vi "SignalGenerator.vi"() -> ()   [LabVIEW 2016]
doc: "I. Description:\nThis example demonstrates how to continuously output a waveform using an internal sample clock. The automatic regeneration of data has been disabled, so new data has to be provided throughout the duration of the continuous Analog Output operation. This allows the generation of any arbitrary frequency as this VI computes new data for each iteration of the loop, maintaining phase continuity of the signal. The regeneration of data has also been adjusted so that the newest data is output as quickly as possible; thus reducing the lag between the changing of the data and the output of that data.\n\nII. Instructions for Running:\n1. Select the Physical Channel to correspond to where your signal is output on the DAQ device.\n2. Enter the Minimum and Maximum Voltage range.\n3. Specify the desired Sample Clock Rate of the output Waveform. Higher sample clock rates will produce a smoother waveform.\n4. Manually specify the Analog Output buffer size, in number of samples. A larger buffer would help non-regenerative operations avoid errors due to occasional high CPU load. \nNote: \nThe Analog Output buffer has to be at least as big as the amount of data being written to the board per iteration. The recommended buffer size would be at least twice the amount of data being written to the board per iteration.\n5. Enter the Waveform Information. See the documentation of the Basic Function Generator SubVI for information on each parameter.\n\nIII. Block Diagram Steps:\n1. Create an Analog Output Voltage channel.\n2. Configure the task to prohibit the automatic regeneration of data.\n2a. Set the transfer condition to Less than Full. Allows for more rapid updates of Output Buffer.\n3. Call the DAQmx (Sample Clock) VI to set the sample clock rate. Additionally, set the sample mode to Continuous.\n4. Read the actual sample clock rate (eventually coerced depending on the hardware used). \n5. Compute the desired waveform, using the buffer size and the actual update rate. This VI keeps track of the phase of the waveform to ensure that the generated signal is continuous.\n6. Write the waveform to the output buffer. \n7a. Call the Start VI. This is only needed when the loop is executed for the first time.\n7b. Do nothing.\n8. Loop continuously until user presses the Stop button. Every iteration computes and writes a new waveform to the buffer.\n9. Call the Clear Task VI to clear the Task.\n10. Use the popup dialog box to display an error or warning if any.\n\nIV. I/O Connections Overview:\nMake sure your signal output terminal matches the Physical Channel I/O Control. For further connection information, refer to your hardware reference manual."
uses:
  <vilib>/Utility/error.llb/DialogType.ctl
  <vilib>/DAQmx/write.llb/DAQmx Write.vi
  <vilib>/DAQmx/create/channels.llb/DAQmx Create Virtual Channel.vi
  <vilib>/DAQmx/configure/timing.llb/DAQmx Timing.vi
  <vilib>/DAQmx/miscellaneous.llb/DAQmx Fill In Error Info.vi
  <vilib>/measure/NI_MABase.lvlib
  <resource>/objmgr/daqmx.rc
panel:
  in  "Size (Samples)":u32=10000
  out "Actual Sample Clock Rate":dbl=20000.0 format="%.2f"
  in  "Sample Clock Rate":dbl=10000.0 format="%0.2f"
  in  "Waveform Type":T1(ring)
  in  "Frequency":dbl=10.0 format="%.2f"
  in  "Amplitude":dbl=0.1 format="%0.2p"
  out "Waveform Graph":waveform(dbl)(graph)={"t0"=timestamp(12.75 s since 1904-01-01), "dt"=5e-05, "Y"=[]} caption="Output Waveform"
  in  "Physical Channels":tag="DAQ/ao0"
  in  "Minimum Value":dbl=-1.0 format="%0.2f"
  in  "Maximum Value":dbl=1.0 format="%0.2f"
  in  "stop":bool
  # "For instructions, select Help>>Show Context Help"
  # "Channel Parameters"
  # "Timing Parameters"
  # "Buffer Parameters"
  # "Waveform Information"
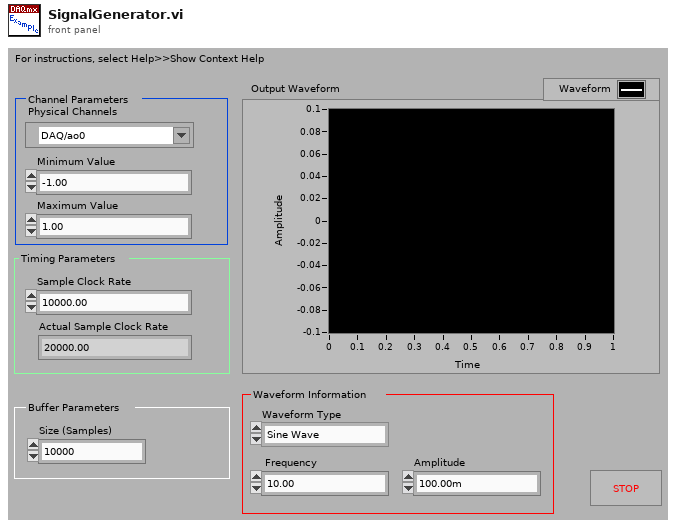
[diagram p1: front panel]
types:
  T1 = enum16{"Sine Wave", "Triangle Wave", "Square Wave", "Sawtooth Wave"}
  T2 = typedef "DialogType.ctl" = u16
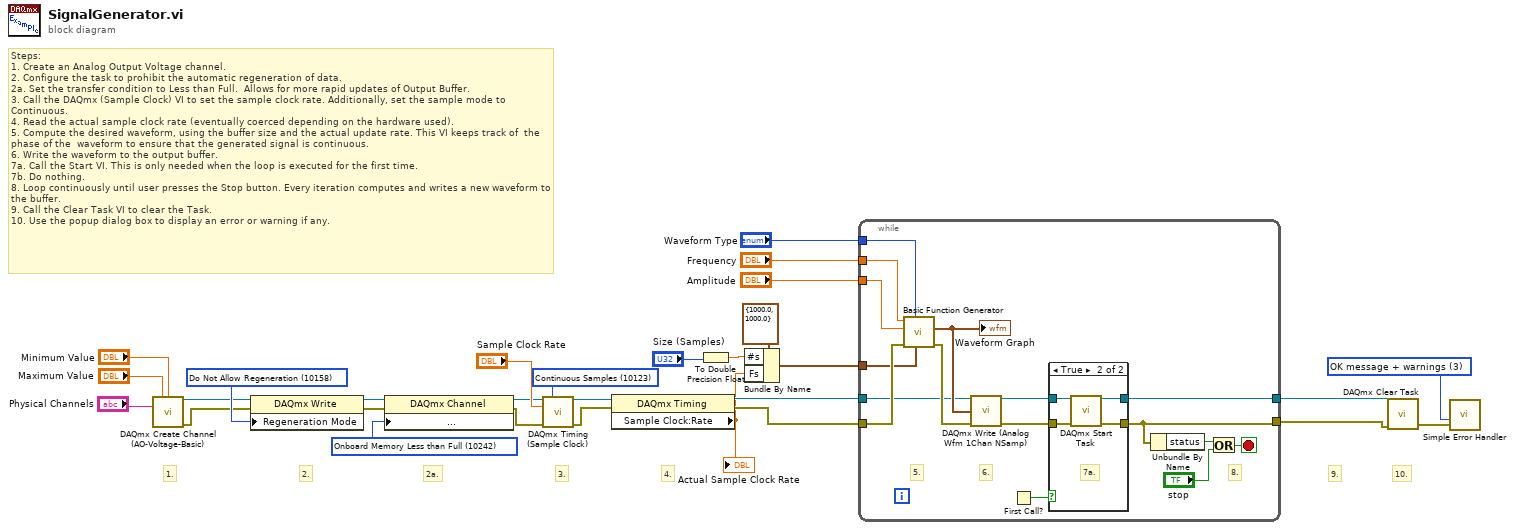
[diagram p0: block diagram]
diagram:
  w6 = 10242 items=["Onboard Memory Empty"=10235, "Onboard Memory Half Full or Less"=10239, "Onboard Memory Less than Full"=10242] ("AO.DataXferReqCond")
  w16 = 10158 items=["Allow Regeneration"=10097, "Do Not Allow Regeneration"=10158] ("RegenMode")
  w24 = T2 3 items=["no dialog", "OK message", "continue or stop message", "OK message + warnings", "continue/stop + warnings"] ("type of dialog (OK msg:1)")
  w28 = 10123 items=["Finite Samples"=10178, "Continuous Samples"=10123] ("sample mode")
  # "2a."
  # "4."
  # "3."
  # "Steps:\n1. Create an Analog Output Voltage channel.\n2. Configure the task to prohibit the automatic regeneration of data.\n2a. Set the transfer condition to Less than Full.  Allows for more rapid updates of Output Buffer. \n3. Call the DAQmx (Sample Clock) VI to set the sample clock rate. Additionally, set the sample mode to Continuous.\n4. Read the actual sample clock rate (eventually coerced depending on the hardware used).\n5. Compute the desired waveform, using the buffer size and the actual update rate. This VI keeps track of  the phase of the  waveform to ensure that the generated signal is continuous.\n6. Write the waveform to the output buffer. \n7a. Call the Start VI. This is only needed when the loop is executed for the first time.\n7b. Do nothing.\n8. Loop continuously until user presses the Stop button. Every iteration computes and writes a new waveform to the buffer.\n9. Call the Clear Task VI to clear the Task.\n10. Use the popup dialog box to display an error or warning if any."
  # "10."
  # "9."
  # "2."
  # "1."
  n1 = call-poly <vilib>:"DAQmx Create Channel (AO-Voltage-Basic).vi"("maximum value"="Maximum Value", "minimum value"="Minimum Value", "physical channels"="Physical Channels") -> ("task out"=w15:refnum<k21>, "error out"=w14:errorcluster)  [unwired: 11 in]
  n2 = property class="DAQmx Write"(reference=w15, error in=w14, "Regeneration Mode"=w16) -> (reference out=w10:refnum<k21>, error out=w7:errorcluster)
  n3 = property class="DAQmx Channel"(reference=w10, error in=w7, "Analog Output:General Properties:Advanced:Data Transfer and Memory:Data Transfer Request Condition"=w6) -> (reference out=w9:refnum<k21>, error out=w8:errorcluster)
  n4 = call-poly <vilib>:"DAQmx Timing (Sample Clock).vi"("task/channels in"=w9, "sample mode"=w28, "rate"="Sample Clock Rate", "error in"=w8) -> ("task out"=w21:refnum<k21>, "error out"=w20:errorcluster)  [unwired: 10 in]
  n5 = property class="DAQmx Timing"(reference=w21, error in=w20) -> (reference out=w4:refnum<k21>, error out=w3:errorcluster, "Sample Clock:Rate"=w1:dbl)
  "Actual Sample Clock Rate" <- w1
  n6 = To Double Precision Float(number="Size (Samples)") -> (double precision float=w11:dbl)
  n7 = Bundle By Name(cluster=cluster{"Fs":dbl, "#s":dbl} {"Fs"=1000.0, "#s"=1000.0} ("sampling info"), "#s"=w11, "Fs"=w1) -> (w5:cluster{"Fs":dbl, "#s":dbl})
  n8 = while {
    tunnel: w4 -> [w35]
    tunnel: [w31] -> w23
    tunnel: w3 -> [w42]
    tunnel: [w32] -> w2
    tunnel: "Waveform Type" -> [w40]
    tunnel: "Frequency" -> [w39]
    tunnel: "Amplitude" -> [w38]
    tunnel: w5 -> [w37]
    stop <- w45 stop-if-true
    # "8."
    # "6."
    # "5."
    n9 = call <vilib>:"Basic Function Generator.vi"("sampling info"=w37, "signal type"=w40, "error in (no error)"=w42, "amplitude"=w38, "frequency"=w39) -> ("error out"=w41:errorcluster, "signal out"=w36:waveform(dbl))  [unwired: 4 in, 1 out]
    "Waveform Graph" <- w36
    n10 = call-poly <vilib>:"DAQmx Write (Analog Wfm 1Chan NSamp).vi"("task/channels in"=w35, "data"=w36, "error in"=w41) -> ("task out"=w34:refnum<k21>, "error out"=w33:errorcluster)  [unwired: 10 in, 1 out]
    n11 = First Call?() -> (First Call?: T/F=w30:bool)
    n12 = case shown="True" w30 {
      tunnel: w34 -> [w47 w51]
      tunnel: w33 -> [w46 w50]
      tunnel: [w46 w49] -> w32
      tunnel: [w47 w48] -> w31
      frame False {
        # "7b."
      }
      frame True {
        # "7a."
        n13 = call <vilib>:"DAQmx Start Task.vi"("task/channels in"=w51, "error in"=w50) -> ("task out"=w48:refnum<k21>, "error out"=w49:errorcluster)  [unwired: 12 in]
      }
    }
    n14 = Unbundle By Name(w32) -> ("status"=w44:bool)
    n15 = Or(x=w44, y="stop") -> (x .or. y?=w45:bool)
  }
  n16 = call <vilib>:"DAQmx Clear Task.vi"("task in"=w23, "error in"=w2) -> ("error out"=w29:errorcluster)  [unwired: 13 in]
  n17 = call <vilib>:"Simple Error Handler.vi"("type of dialog (OK msg:1)"=w24, "error in (no error)"=w29) -> ()  [unwired: 3 in, 5 out]
